vi "Test.vi"() -> ()   [LabVIEW 2021]
uses:
  <vilib>/NI/LVFPGA Adv Session Resources/ResourceInfo.ctl
  <vilib>/NI/LVFPGA Adv Session Resources/OpenByNameSubVI.vi
  <vilib>/FPGAPlugInAG/cRIO-9053/niLvFpga_Open_cRIO-9053.vi
  <vilib>/rvi/interface/common/dynamic/niFpgaDynamicAddResources.vi
  <vilib>/rvi/interface/common/dynamic/niFpgaEscapeDelimiterAndNull.vi
  <vilib>/Utility/error.llb/Error Cluster From Error Code.vi
  <vilib>/rvi/errors/niLvFpgaAdjustHostInterfaceError.vi
  <vilib>/FPGAPlugInAG/Dynamic/niLvFpga_Close_Dynamic.vi
  <vilib>/rvi/interface/nirviOpenFPGA/nirviOpenFPGA.xnode
  FPGA Bitfiles/fpga-bus_FPGATarget_ExampleFPGAMain.lvbitx
  <vilib>/NI/LVFPGA Adv Session Resources/OpenByName.xnode
  <vilib>/rvi/interface/nirviReadWriteControl/nirviReadWriteControl.xnode
  <vilib>/rvi/interface/nirviCloseFPGA/nirviCloseFPGA.xnode
  <vilib>/NI/LVFPGA Adv Session Resources/LVFPGAAdvSessionResources.lvlib
  NiFpgaLv.dll
  <vilib>/rvi/interface/Simulation/niFpgaSimulationCallBeginRW.vi
panel:
  in  "stop":bool
  out "Value 2":i16
  out "Error out 2":errorcluster
  in  "Value":i16
  out "Error out":errorcluster
  out "Resource info out":T1[](array[typedef])
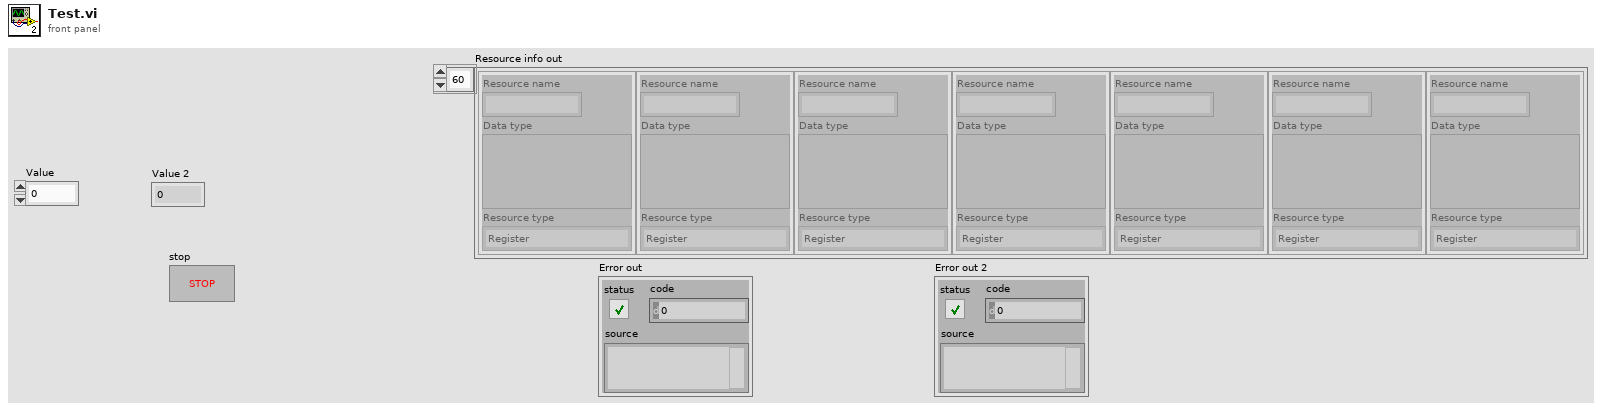
[diagram p1: front panel]
types:
  T1 = typedef "LVFPGAAdvSessionResources.lvlib/ResourceInfo.ctl" = cluster{"Resource name":string, "Data type":variant, "Resource type":enum16{"Register", "Host To Target FIFO", "Target To Host FIFO"}}
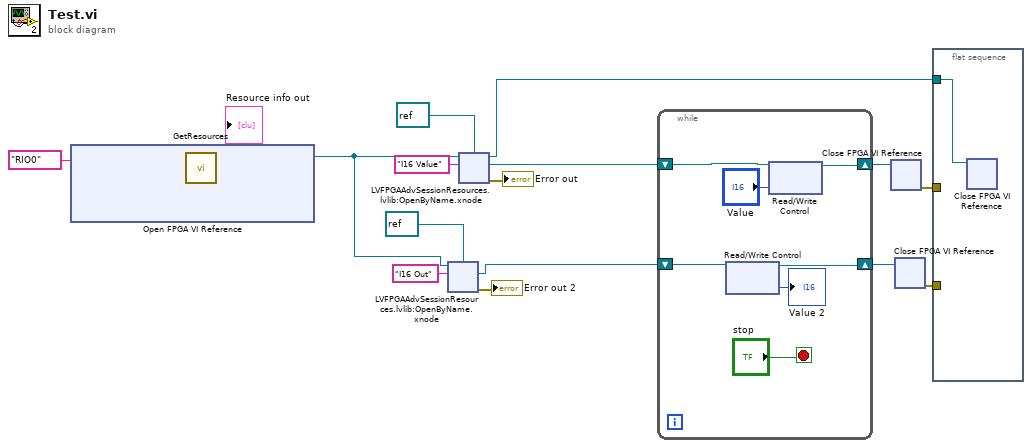
[diagram p0: block diagram]
diagram:
  n1 = xnode "Open FPGA VI Reference"("resource name"=tag "RIO0") -> ("FPGA VI Reference Out"=w14:refnum<k20>)  [unwired: 1 in, 1 out]
  n2 = call <vilib>:"GetResources.vi"("FPGA VI Reference in"=w14) -> ("Resource info out"=→"Resource info out":T1[], "FPGA VI Reference out"=w1:refnum<k20>)  [unwired: 8 in, 1 out]
  n3 = xnode "LVFPGAAdvSessionResources.lvlib:OpenByName.xnode"("FPGA VI Reference in"=w1, "Resource name in"="I16 Out", "Single resource reference type in"=refnum<k20> refnum ("FPGA Interface")) -> ("Single resource reference out"=w2:refnum<k20>, "Error out"=→"Error out 2":errorcluster)  [unwired: 1 in, 1 out]
  n4 = xnode "LVFPGAAdvSessionResources.lvlib:OpenByName.xnode"("FPGA VI Reference in"=w1, "Resource name in"="I16 Value", "Single resource reference type in"=refnum<k20> refnum ("FPGA Interface")) -> ("Single resource reference out"=w10:refnum<k20>, "Error out"=→"Error out":errorcluster, "FPGA VI Reference out"=w16:refnum<k20>)  [unwired: 1 in]
  n5 = while {
    shift-right: [w22] -> w6
    shift-left: w10 -> [w24]
    shift-right: [w20] -> w5
    shift-left: w2 -> [w21]
    stop <- "stop" stop-if-true
    n6 = xnode "Read/Write Control"("FPGA VI Reference In"=w21) -> ("FPGA VI Reference Out"=w20:refnum<k20>, "Value"=→"Value 2":i16)  [unwired: 1 in, 1 out]
    n7 = xnode "Read/Write Control"("FPGA VI Reference In"=w24, "Value"="Value") -> ("FPGA VI Reference Out"=w22:refnum<k20>)  [unwired: 1 in, 1 out]
  }
  n8 = xnode "Close FPGA VI Reference"("FPGA VI Reference In"=w6) -> ("error out"=w4:errorcluster)  [unwired: 1 in]
  n9 = xnode "Close FPGA VI Reference"("FPGA VI Reference In"=w5) -> ("error out"=w3:errorcluster)  [unwired: 1 in]
  n10 = flat-sequence {
    tunnel: w16 -> [w25]
    tunnel: w4 -> [_]
    tunnel: w3 -> [_]
    frame #0 {
      n11 = xnode "Close FPGA VI Reference"("FPGA VI Reference In"=w25) -> ()  [unwired: 1 in, 1 out]
    }
  }
